vi "setUp.vi"(8 "error in (no error)":errorcluster, 11 "reference in":refnum<class "testcase-Basic-Function.lvclass">) -> (0 "error out":errorcluster, 3 "reference out":refnum<class "testcase-Basic-Function.lvclass">)   [LabVIEW 2017, in "testcase-Basic-Function.lvclass"]
doc: "setUp runs prior to the test method during test execution. Use this method to initialize any object data required by your tests."
uses:
  testcase-Basic-Function.lvclass
  C:/Program Files (x86)/National Instruments/LabVIEW 2017/vi.lib/addons/_JKI Toolkits/VI Tester/TestCase.llb/TestCase.lvclass
  testcase-Basic-Function.lvclass/testcase-Basic-Function.ctl
  <vilib>/addons/_JKI Toolkits/VI Tester/TestCase.llb/TestCase.lvclass
  src/examples/NEVSTOP/Communicable State Machine(CSM)/1. Create a reuse Module/1. Create a reuse Module.lvlib
  src/user.lib/_NEVSTOP/Communicable State Machine(CSM)/Communicable State Machine.lvlib
  CSM/CSM-Testcase.lvlib
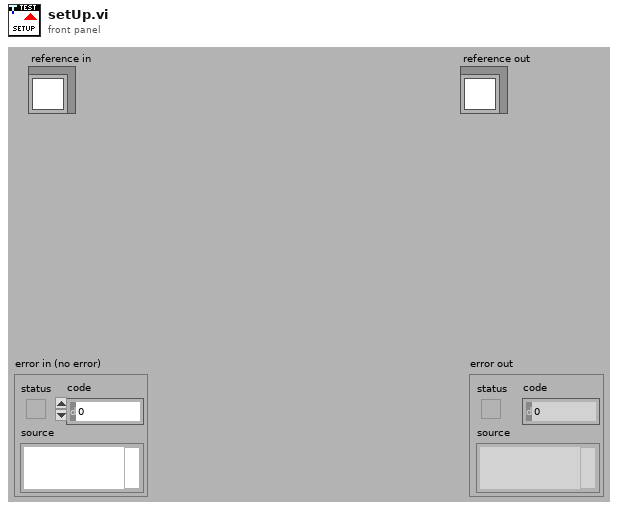
[diagram p1: front panel]
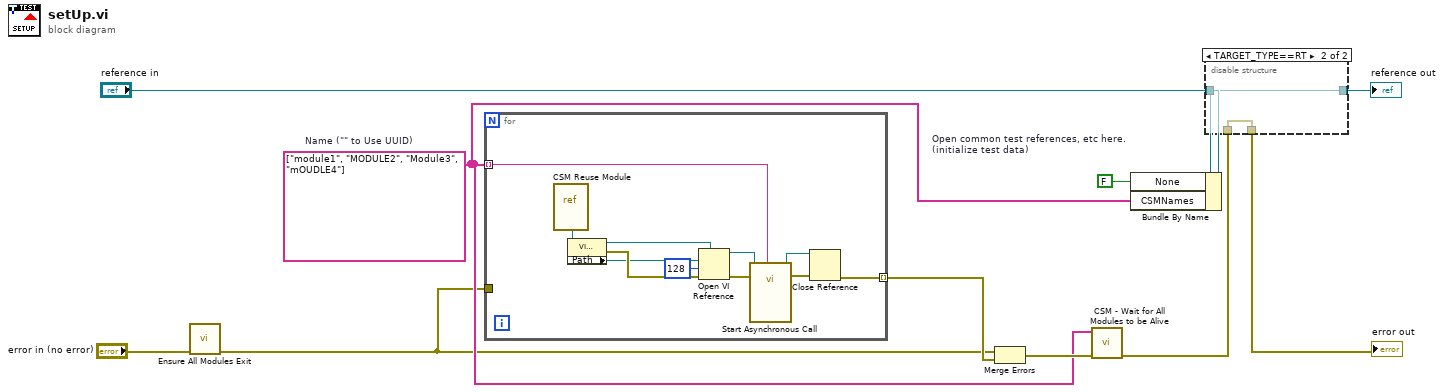
[diagram p0: block diagram]
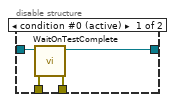
[diagram p2: hidden frame]
diagram:
  w2 = string[] ["module1", "MODULE2", "Module3", "mOUDLE4"]  # Name ("" to Use UUID)
  w6 = FALSE  # Open common test references, etc here. (initialize test data)
  n1 = call "Ensure All Modules Exit.vi"("Error in"="error in (no error)") -> ("Error out"=w1:errorcluster)  [unwired: 10 in]
  n2 = for {
    tunnel: w2 -> [w19] mode=indexing
    tunnel: [w12] -> w4 mode=indexing
    tunnel: w1 -> [_]
    n3 = vi-ref "CSM Reuse Module.vi"() -> (w14:refnum<vi>)
    n4 = property class="VI (strict)"(reference=w14) -> (reference out=w18:refnum<vi>, error out=w16:errorcluster, "Path"=w15:path)  [unwired: 1 in]
    n5 = Open VI Reference(type specifier VI Refnum (for type only)=w18, vi path=w15, options=128, error in (no error)=w16) -> (vi reference=w17:refnum<vi>, error out=w13:errorcluster)  [unwired: 2 in]
    n6 = call-by-ref "Start Asynchronous Call"(reference=w17, error in=w13, "Name(\"\" to use uuid)"=w19) -> (reference out=w21:refnum<vi>, error out=w20:errorcluster)  [unwired: 11 in]
    n7 = Close Reference(reference=w21, error in (no error)=w20) -> (error out=w12:errorcluster)
  }
  n8 = Merge Errors(w1, w4) -> (w5:errorcluster)
  n9 = call "CSM - Wait for All Modules to be Alive.vi"("Error In"=w5, "CSM Names"=w2) -> ("error out"=w3:errorcluster)  [unwired: 7 in, 2 out]
  n10 = Bundle By Name(cluster="reference in", "None"=w6, "CSMNames"=w2) -> (w7:refnum<class "testcase-Basic-Function.lvclass">)
  n11 = disable-structure shown="TARGET_TYPE==RT" {
    disable-tunnel: w3 -> [w26 w27]
    disable-tunnel: [w25 w27] -> w10
    disable-tunnel: [w24 w28] -> w8
    disable-tunnel: w7 -> [w23 w28]
    frame condition #0 (active) {
      n12 = call <vilib>:"WaitOnTestComplete.vi"("error in (no error)"=w26, "TestCase in"=w23) -> ("error out"=w25:errorcluster, "TestCase out"=w24:refnum<class "testcase-Basic-Function.lvclass">)  [unwired: 8 in]
    }
    frame condition #1 {
    }
  }
  "error out" <- w10
  "reference out" <- w8
